vi "Write reader.vi"(10 "reader":refnum<k21>, 11 "Network Stream in":refnum<class "Network Stream.lvclass">) -> (3 "Network Stream out":refnum<class "Network Stream.lvclass">)   [LabVIEW 2020, in "Network Stream.lvclass"]
uses:
  Network Stream.lvclass
  Network Stream.lvclass/Network Stream.ctl
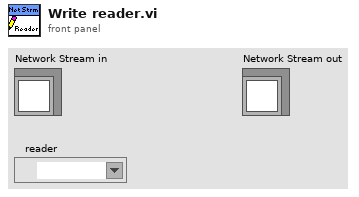
[diagram p1: front panel]
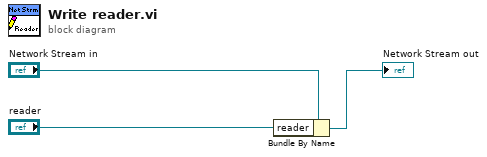
[diagram p0: block diagram]
diagram:
  n1 = Bundle By Name(cluster="Network Stream in", "reader"="reader") -> (→"Network Stream out":refnum<class "Network Stream.lvclass">)
